vi "DP mode ring to Text.vi"(1 "Mode":enum16{"L1 = L2", "L1 = L2 + 10 dB"}(ring)) -> (0 "Text":string)   [LabVIEW 2020]
panel:
  in  "Waveform":i32(ring) items=["TONE PIP", "CLICK"]
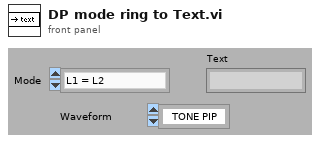
[diagram p1: front panel]
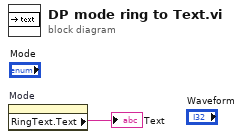
[diagram p0: block diagram]
diagram:
  n1 = property on="Mode" class="Enum (strict)"() -> ("RingText.Text"=→"Text":string)  [unwired: 2 in, 2 out]
